vi "WaitForStateChange.vi"(8 "error in (no error)":errorcluster, 9 "timeout in ms (-1)":i32=-1, 10 "State (unknown: Any state change)":T1, 11 "SMO in":refnum<class "SMO.lvclass">) -> (0 "error out":errorcluster, 1 "timed out":bool, 3 "SMO out":refnum<class "SMO.lvclass">)   [LabVIEW 2013, in "SMO.lvclass"]
uses:
  SMO.lvclass
  Typedefs/SMOState --Enum.ctl
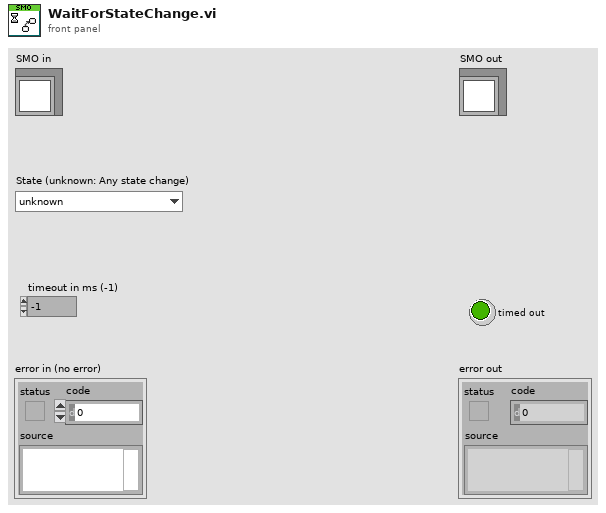
[diagram p1: front panel]
types:
  T1 = typedef "SMO.lvclass/SMOState --Enum.ctl" = enum16{"unknown", "Created", "Started", "Stopped"}
  T2 = typedef "SMO.lvclass/Protected Events.ctl" = cluster{"StopProcesses":refnum<user-event>, "AbortProcesses":refnum<user-event>, "Config Changed":refnum<user-event>}
  T3 = typedef "SMO.lvclass/Public Events.ctl" = cluster{"Error":refnum<user-event>, "State":refnum<user-event>}
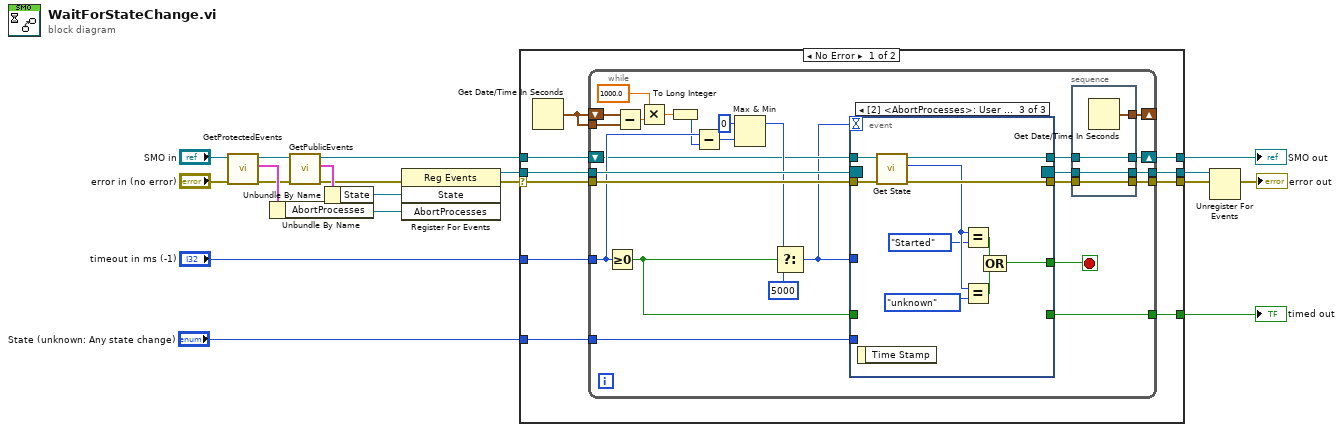
[diagram p0: block diagram]
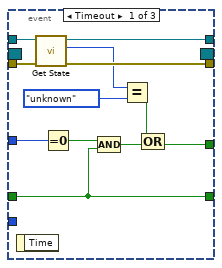
[diagram p2: hidden frame]
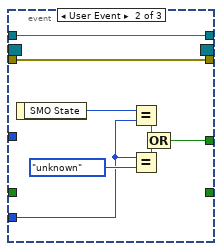
[diagram p3: hidden frame]
diagram:
  n1 = call "GetProtectedEvents.vi"("error in (no error)"="error in (no error)", "SMO"="SMO in") -> ("error out"=w6:errorcluster, "SMO Protected Events"=w10:T2, "SMO out"=w8:refnum<class "SMO.lvclass">)  [unwired: 7 in]
  n2 = Unbundle By Name(w10) -> ("AbortProcesses"=w11:refnum<user-event>)
  n3 = call "GetPublicEvents.vi"("error in (no error)"=w6, "SMO"=w8) -> ("error out"=w5:errorcluster, "Public Events"=w9:T3, "SMO out"=w7:refnum<class "SMO.lvclass">)  [unwired: 7 in]
  n4 = Unbundle By Name(w9) -> ("State"=w15:refnum<user-event>)
  n5 = register-events(error in=w5, w15, w11) -> (reference out=w14:refnum<event-registration>, error out=w16:errorcluster)  [unwired: 1 in]
  n6 = case shown="No Error" w16 {
    selector: w16 -> [w27 w92]
    tunnel: [w29 w92] -> w2
    tunnel: w14 -> [w28 w91]
    tunnel: "timeout in ms (-1)" -> [w26 _]
    tunnel: [w25 w91] -> w17
    tunnel: "State (unknown: Any state change)" -> [w24 _]
    tunnel: [w23 _] -> w13
    tunnel: w7 -> [w22 w90]
    tunnel: [w21 w90] -> w12
    frame No Error {
      n7 = Get Date/Time In Seconds() -> (seconds since 1Jan1904=w20:timestamp)
      n8 = while {
        tunnel: [w32] -> w29
        tunnel: w28 -> [w55]
        tunnel: w27 -> [w54]
        tunnel: w26 -> [w43]
        tunnel: [w33] -> w25
        tunnel: w24 -> [w53]
        shift-right: [w47] -> _
        shift-left: w20 -> [w46]
        tunnel: [w49] -> w23
        shift-right: [w35] -> w21
        shift-left: w22 -> [w38]
        tunnel: w20 -> [w45]
        stop <- w30 stop-if-true
        n9 = Greater Or Equal To 0?(x=w43) -> (x >= 0?=w48:bool)
        n10 = Subtract(x=w46, y=w45) -> (x-y=w44:dbl)
        n11 = Multiply(x=1000.0 ("timeout in ms (-1)"), y=w44) -> (x*y=w50:dbl)
        n12 = To Long Integer(number=w50) -> (32bit integer=w42:i32)
        n13 = Subtract(x=w43, y=w42) -> (x-y=w41:i32)
        n14 = Max & Min(x=0, y=w41) -> (max(x,y)=w39:i32)  [unwired: 1 out]
        n15 = Select(t=w39, s=w48, f=5000 ("timeout in ms (-1)")) -> (s? t:f=w37:i32)
        n16 = event shown="[2] <AbortProcesses>: User Event" {
          selector: w55 -> [_ _ _]
          dyn-events: [_ _ _] -> w34
          timeout: w37 -> [_ _ _]
          tunnel: w54 -> [w67 w79 w87]
          tunnel: [w66 w79 w86] -> w31
          tunnel: [w69 w72 w80] -> w30
          tunnel: w53 -> [_ w74 _]
          tunnel: [w60 _ _] -> w49
          tunnel: w48 -> [w60 _ _]
          tunnel: w37 -> [w62 _ _]
          tunnel: w38 -> [w71 w73 w89]
          tunnel: [w70 w73 w88] -> w36
          event Timeout {
            n17 = event-data() -> ()  [unwired: 1 in, 1 out]
            n18 = call "Get State.vi"("error in (no error)"=w67, "SMO"=w71) -> ("error out"=w66:errorcluster, "SMO State"=w64:T1, "SMO out"=w70:refnum<class "SMO.lvclass">)  [unwired: 7 in]
            n19 = Equal To 0?(x=w62) -> (x = 0?=w61:bool)
            n20 = Compound Arithmetic op=AND(w61, w60) -> (w63:bool)
            n21 = Equal?(x=w64, y=SMOState_--Enum."unknown") -> (x = y?=w68:bool)
            n22 = Compound Arithmetic op=OR(w68, w63) -> (w69:bool)
          }
          event User Event {
            n23 = event-data() -> ("SMO State"=w76:T1)  [unwired: 1 in]
            n24 = Equal?(x=w76, y=w74) -> (x = y?=w77:bool)
            n25 = Equal?(x=w74, y=SMOState_--Enum."unknown") -> (x = y?=w78:bool)
            n26 = Compound Arithmetic op=OR(w77, w78) -> (w72:bool)
          }
          event User Event {
            n27 = event-data() -> ()  [unwired: 1 in, 1 out]
            n28 = call "Get State.vi"("error in (no error)"=w87, "SMO"=w89) -> ("error out"=w86:errorcluster, "SMO State"=w84:T1, "SMO out"=w88:refnum<class "SMO.lvclass">)  [unwired: 7 in]
            n29 = Equal?(x=w84, y=SMOState_--Enum."Started") -> (x = y?=w82:bool)
            n30 = Equal?(x=w84, y=SMOState_--Enum."unknown") -> (x = y?=w81:bool)
            n31 = Compound Arithmetic op=OR(w82, w81) -> (w80:bool)
          }
        }
        n32 = stacked-sequence {
          tunnel: [w59] -> w47
          tunnel: w36 -> [w58]
          tunnel: [w58] -> w35
          tunnel: w34 -> [w57]
          tunnel: [w57] -> w33
          tunnel: [w56] -> w32
          tunnel: w31 -> [w56]
          frame #0 {
            n33 = Get Date/Time In Seconds() -> (seconds since 1Jan1904=w59:timestamp)
          }
        }
      }
    }
    frame Error {
    }
  }
  "SMO out" <- w12
  "timed out" <- w13
  n34 = Unregister For Events(event registration refnum=w17, error in=w2) -> (error out=→"error out":errorcluster)
